vi "Run Bfr Rx - Cached - Flush Cache.vi"(5 "Cache Buffer":u64 format="%016x", 8 "error in (no error)":errorcluster, 11 "Null Data in":u8[](array[numeric])) -> (0 "error out":errorcluster)   [LabVIEW 2021, in "UDP-Custom-Device Engine.lvlib"]
uses:
  UDP-Custom-Device Engine.lvlib
  <vilib>/NI VeriStand/VeriStand Data/Pointer Operations/Pointer.Write (1D U8).vi
  <vilib>/NI VeriStand/VeriStand Data/VeriStand Data.lvlib
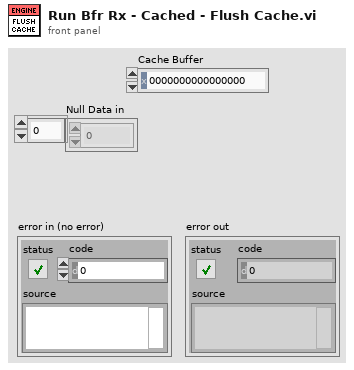
[diagram p1: front panel]
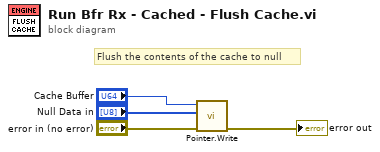
[diagram p0: block diagram]
diagram:
  # "Flush the contents of the cache to null"
  n1 = call-poly <vilib>:"Pointer.Write.vi"("error in (no error)"="error in (no error)", "values"="Null Data in", "pointer in"="Cache Buffer") -> ("error out"=→"error out":errorcluster)  [unwired: 6 in, 2 out]
